vi "ResonanceAnalyzerJ&J.vi"() -> ()   [LabVIEW 2015]
uses:
  <vilib>/imath/engines/lvmath/Plug In/_Char/NIMS_CH_character datatype.ctl
  <vilib>/imath/engines/lvmath2/RunTimeEngine/Managers/WorkSpace/UID Generator.vi
  <vilib>/imath/engines/lvmath2/RunTimeEngine/RunTimeType/NIMS_RunTimeType_From StrictType (excl LVString).vi
  <instcachedir>/0/NIMS_RunTimeType_From StrictType (excl LVString)_EB1C38A9BC5048DA9ABDA8F781E54D21.lvgen/NIMS_RunTimeType_From StrictType (excl LVString)_EB1C38A9BC5048DA9ABDA8F781E54D21_000.vi
  <vilib>/imath/engines/lvmath2/RunTimeEngine/LocalVariableDefStatement/MC_LocalVariableDefStatement_Display.vi
  <vilib>/imath/engines/lvmath2/RunTimeEngine/BuiltInFunctions/linramp/NIMS_linramp.vi
  <vilib>/imath/engines/lvmath2/RunTimeEngine/ArithmeticOperatorToken/NIMS_ArithmeticOperator_minus.vi
  <instcachedir>/0/NIMS_ArithmeticOperator_minus_8228ED1EA52B4CB8A68367813E4B0C9D.lvgen/NIMS_ArithmeticOperator_minus_8228ED1EA52B4CB8A68367813E4B0C9D_003.vi
  <vilib>/imathl/engines/lvmath/Functions/Error Handling/Create Error.vi
  <vilib>/imath/engines/lvmath2/RunTimeEngine/ArithmeticOperatorToken/NIMS_ArithmeticOperator_times.vi
  <instcachedir>/0/NIMS_ArithmeticOperator_times_DF26C4080E2A467BA28C929B8CF31953.lvgen/NIMS_ArithmeticOperator_times_DF26C4080E2A467BA28C929B8CF31953_000.vi
  <vilib>/imath/engines/lvmath/Plug In/_Char/NIMS_CH_Character RV to String.vi
  <vilib>/imath/engines/lvmath2/RunTimeEngine/BuiltInFunctions/random/NIMS_random.vi
  <vilib>/imath/engines/lvmath2/RunTimeEngine/IndexRead/NIMS M(S).vi
  <instcachedir>/0/NIMS M(S)_B826C018497E4940AE96BD27B540B6FB.lvgen/NIMS M(S)_B826C018497E4940AE96BD27B540B6FB_000.vi
  <vilib>/imath/engines/lvmath2/RunTimeEngine/Managers/SymbolTable/Clear UID.vi
  <vilib>/imath/engines/lvmath2/RunTimeEngine/NodeEndStatement/NIMS_NodeEndStatement_Output.vi
  <instcachedir>/0/NIMS_NodeEndStatement_Output_53EC0D466D134D7ABD903AC30B43404B.lvgen/NIMS_NodeEndStatement_Output_53EC0D466D134D7ABD903AC30B43404B_005.vi
  <vilib>/imath/engines/lvmath2/RunTimeEngine/ErrorHandling/NIMS_Finalize Error.vi
  <vilib>/imath/engines/lvmath2/RunTimeEngine/Managers/SymbolTable/NIMS_WorkSpace.lvlib
panel:
  out "Results":T1
  out "Resonance Curve":cluster{"all rows":dbl[], "Array":dbl[]}[](graph)
  in  "Tab Control":enum32{"Simulation", "Experiment"}(tab)
  in  "Input Parameter":T2
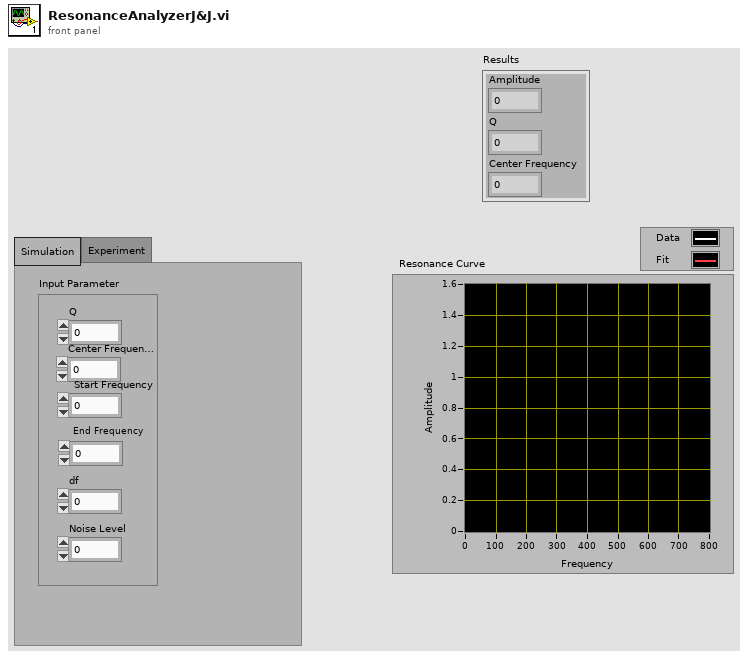
[diagram p1: front panel]
types:
  T1 = cluster{"Amplitude":dbl, "Q":dbl, "Center Frequency":dbl}
  T2 = cluster{"Q":dbl, "Center Frequency":dbl, "Start Frequency":dbl, " End Frequency":dbl, "df":dbl, "Noise Level":dbl}
  T3 = typedef "NIMS_CH_character datatype.ctl" = cluster{"Numeric":u8}
  T4 = cluster{"Array[0]":dbl, "Array[1]":dbl, "Array[2]":dbl, "Array[3]":dbl, "Array[4]":dbl, "Array[5]":dbl, "Array[6]":dbl, "Array[7]":dbl, "Array[8]":dbl}
  T5 = cluster{"Array[0]":dbl, "Array[1]":dbl, "Array[2]":dbl}
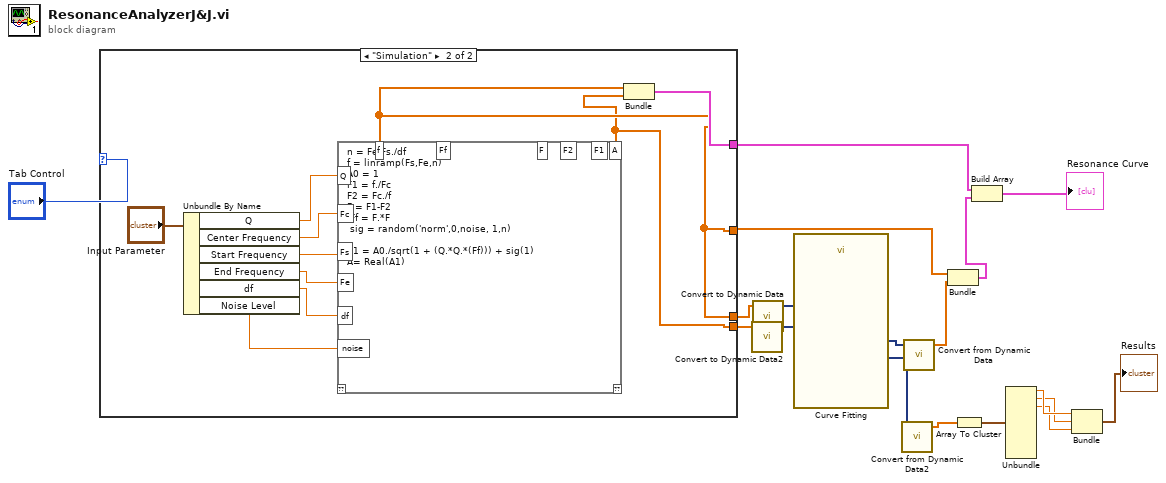
[diagram p0: block diagram]
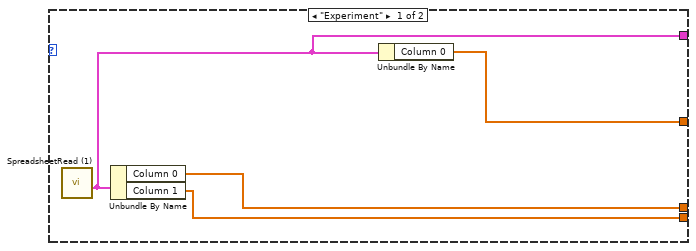
[diagram p2: hidden frame]
diagram:
  n1 = case shown="\"Simulation\"" "Tab Control" {
    tunnel: [w21 w24] -> w9
    tunnel: [w22 w25] -> w18
    tunnel: [w20 w24] -> w13
    tunnel: [w19 w23] -> w12
    frame "Experiment" {
      n2 = call "SpreadsheetRead (1).vi"() -> ("Output Cluster"=w22:cluster{"Column 0":dbl[], "Column 1":dbl[]})  [unwired: 10 in, 1 out]
      n3 = Unbundle By Name(w22) -> ("Column 0"=w20:dbl[], "Column 1"=w19:dbl[])
      n4 = Unbundle By Name(w22) -> ("Column 0"=w21:dbl[])
    }
    frame "Simulation" {
      n5 = Unbundle By Name("Input Parameter") -> ("Q"=w31:dbl, "Center Frequency"=w30:dbl, "Start Frequency"=w29:dbl, "End Frequency"=w28:dbl, "df"=w27:dbl, "Noise Level"=w26:dbl)
      n6 = mathscript code="n = Fe-Fs./df\nf = linramp(Fs,Fe,n)\nA0 = 1\nF1 = f./Fc\nF2 = Fc./f\nF = F1-F2\n Ff = F.*F\n sig = random('norm',0,noise, 1,n)\n\nA1 = A0./sqrt(1 + (Q.*Q.*(Ff))) + sig(1)\nA= Real(A1)"("Q"=w31, "Fc"=w30, "Fs"=w29, "Fe"=w28, "df"=w27, "noise"=w26) -> ("A"=w23:dbl[], "f"=w24:dbl[])  [unwired: 1 in, 5 out]
      n7 = Bundle("f"=w24, "A"=w23) -> (w25:cluster{"f":dbl[], "A":dbl[]})  [unwired: 1 in]
    }
  }
  n8 = call "Convert to Dynamic Data2"("Array"=w12) -> ("Dynamic Data Type"=w11:dynamicdata)  [unwired: 3 in]
  n9 = call "Convert to Dynamic Data"("Array"=w13) -> ("Dynamic Data Type"=w10:dynamicdata)  [unwired: 3 in]
  n10 = call "Curve Fitting"("Locations"=w10, "Signals"=w11) -> ("best fit"=w15:dynamicdata, "non-linear coefficients"=w7:dynamicdata)  [unwired: 5 in, 3 out]
  n11 = call "Convert from Dynamic Data2"("Dynamic Data Type"=w7) -> ("Array"=w6:dbl[])  [unwired: 3 in]
  n12 = call "Convert from Dynamic Data"("Dynamic Data Type"=w15) -> ("Array"=w14:dbl[])  [unwired: 3 in]
  n13 = Bundle("f"=w9, "Array"=w14) -> (w8:cluster{"f":dbl[], "Array":dbl[]})  [unwired: 1 in]
  n14 = Array To Cluster(array=w6) -> (cluster=w5:T4)
  n15 = Build Array(w18, w8) -> (→"Resonance Curve":cluster{"f":dbl[], "Array":dbl[]}[])
  n16 = Unbundle(w5) -> ("Array[0]"=w4:dbl, "Array[1]"=w3:dbl, "Array[2]"=w2:dbl)  [unwired: 6 out]
  n17 = Bundle("Array[0]"=w4, "Array[1]"=w3, "Array[2]"=w2) -> (→"Results":T5)  [unwired: 1 in]
